vi "X_Compensate_Calc.vi"(7 "Angle to Normal":dbl=60.0, 10 "Delta_Z":dbl) -> (2 "Delta_X":dbl)   [LabVIEW 2011]
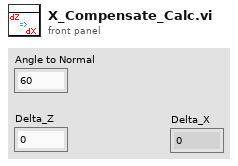
[diagram p1: front panel]
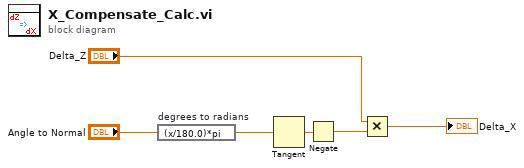
[diagram p0: block diagram]
diagram:
  n1 = expression code="(x/180.0)*pi" "degrees to radians"("Angle to Normal") -> (w5:dbl)
  n2 = Tangent(1:w5) -> (0:w6:dbl)
  n3 = Negate(x=w6) -> (-x=w3:dbl)
  n4 = Multiply(x="Delta_Z", y=w3) -> (x*y=→"Delta_X":dbl)
